vi "RunTests.vi"() -> ()   [LabVIEW 2019]
panel:
  out "Passed?":bool[](array[boolean])
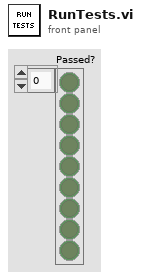
[diagram p1: front panel]
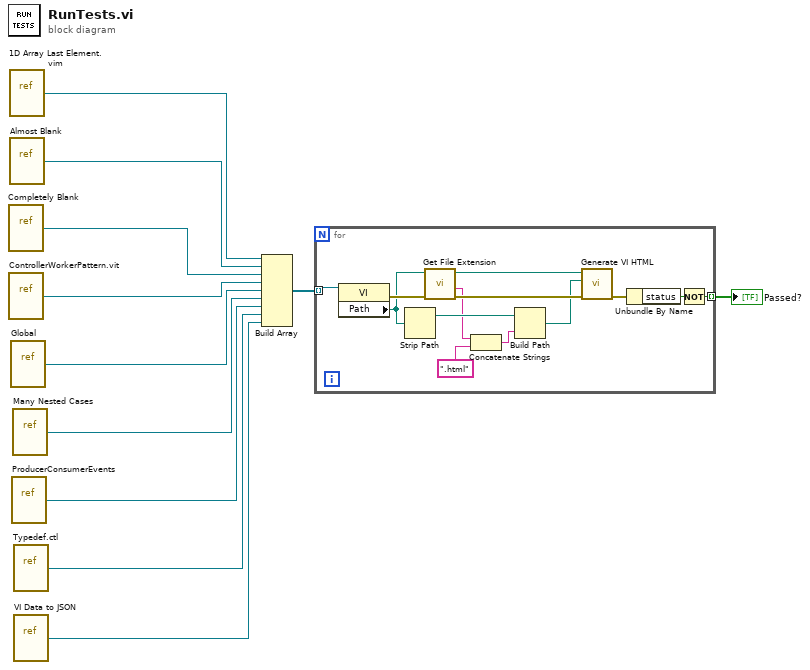
[diagram p0: block diagram]
diagram:
  n1 = vi-ref "Completely Blank.vi"() -> (w10:refnum<vi>)
  n2 = vi-ref "ControllerWorkerPattern.vit"() -> (w9:refnum<vi>)
  n3 = vi-ref "1D Array Last Element.vim"() -> (w2:refnum<vi>)
  n4 = vi-ref "Almost Blank.vi"() -> (w11:refnum<vi>)
  n5 = vi-ref "Global.vi"() -> (w8:refnum<vi>)
  n6 = vi-ref "ProducerConsumerEvents.vi"() -> (w7:refnum<vi>)
  n7 = vi-ref "Many Nested Cases.vi"() -> (w3:refnum<vi>)
  n8 = vi-ref "Typedef.ctl"() -> (w4:refnum<vi>)
  n9 = vi-ref "VI Data to JSON.vi"() -> (w1:refnum<vi>)
  n10 = Build Array(w2, w11, w10, w9, w8, w3, w7, w4, w1) -> (w6:refnum<vi>[])
  n11 = for {
    tunnel: w6 -> [w24] mode=indexing
    tunnel: [w13] -> w5 mode=indexing
    n12 = property class="VI"(reference=w24) -> (error out=w23:errorcluster, "Path"=w20:path)  [unwired: 1 in, 1 out]
    n13 = Strip Path(path=w20) -> (stripped path=w19:path)  [unwired: 1 out]
    n14 = call <vilib>:"Get File Extension.vi"("error in (no error)"=w23, "file"=w20) -> ("error out"=w22:errorcluster, "filename without extension"=w18:string, "dup file"=w21:path)  [unwired: 5 in, 2 out]
    n15 = Concatenate Strings(w18, ".html" ("string")) -> (w16:string)
    n16 = Build Path(base path=w19, name or relative path=w16) -> (appended path=w15:path)
    n17 = call "Generate VI HTML.vi"("error in"=w22, "Output path"=w15, "VI Path"=w21) -> ("error out"=w12:errorcluster)  [unwired: 7 in, 1 out]
    n18 = Unbundle By Name(w12) -> ("status"=w14:bool)
    n19 = Not(x=w14) -> (.not. x?=w13:bool)
  }
  "Passed?" <- w5
